vi "Initialize.vi"(7 "Serial Configuration":T1={"Baud Rate"=9600, "Parity"=0, "Data Bits"=8, "Stop Bits"=10, "Flow Control"=0} {"Flow Control" items=["None", "XON/XOFF", "RTS/CTS", "XON/XOFF & RTS/CTS", "DTR/DSR", "XON/XOFF & DTR/DSR"]; "Stop Bits" items=["1.0"=10, "1.5"=15, "2.0"=20]; "Data Bits" items=["7"=7, "8"=8]; "Parity" items=["None", "Odd", "Even", "Mark", "Space"]; "Baud Rate" items=["300"=300, "600"=600, "1200"=1200, "2400"=2400, "4800"=4800, "9600"=9600, "19200"=19200]}, 8 "error in (no error)":errorcluster, 9 "Reset (True)":bool=TRUE, 10 "ID Query (True)":bool=TRUE, 11 "VISA resource name":refnum<visa-resource-name>) -> (0 "error out":errorcluster, 3 "VISA resource name out":refnum<visa-resource-name>)   [LabVIEW 2012, in "Fluke 5080.lvlib"]
doc: "Establishes communication with the instrument and optionally performs an instrument identification query and/or an instrument reset. It also places the instrument in a default state needed for other instrument driver operations. Therefore, call this VI before calling other instrument driver VIs for this instrument. Generally, you need to call the Initialize VI only once at the beginning of an application."
uses:
  <instrlib>/Fluke 5080/Fluke 5080.lvlib
panel:
  # "(c) 2010 National Instruments.  ALL RIGHTS RESERVED."
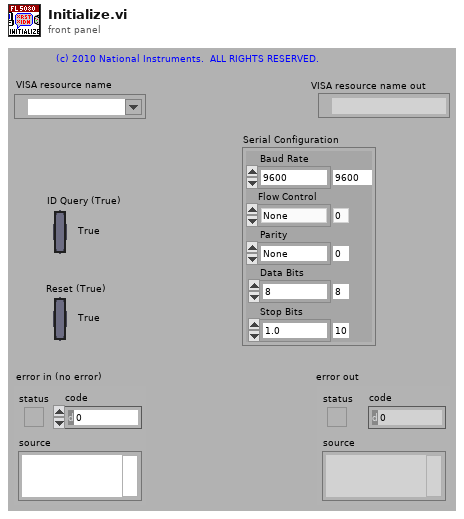
[diagram p1: front panel]
types:
  T1 = cluster{"Baud Rate":u32, "Parity":u16, "Data Bits":u16, "Stop Bits":u16, "Flow Control":u16}
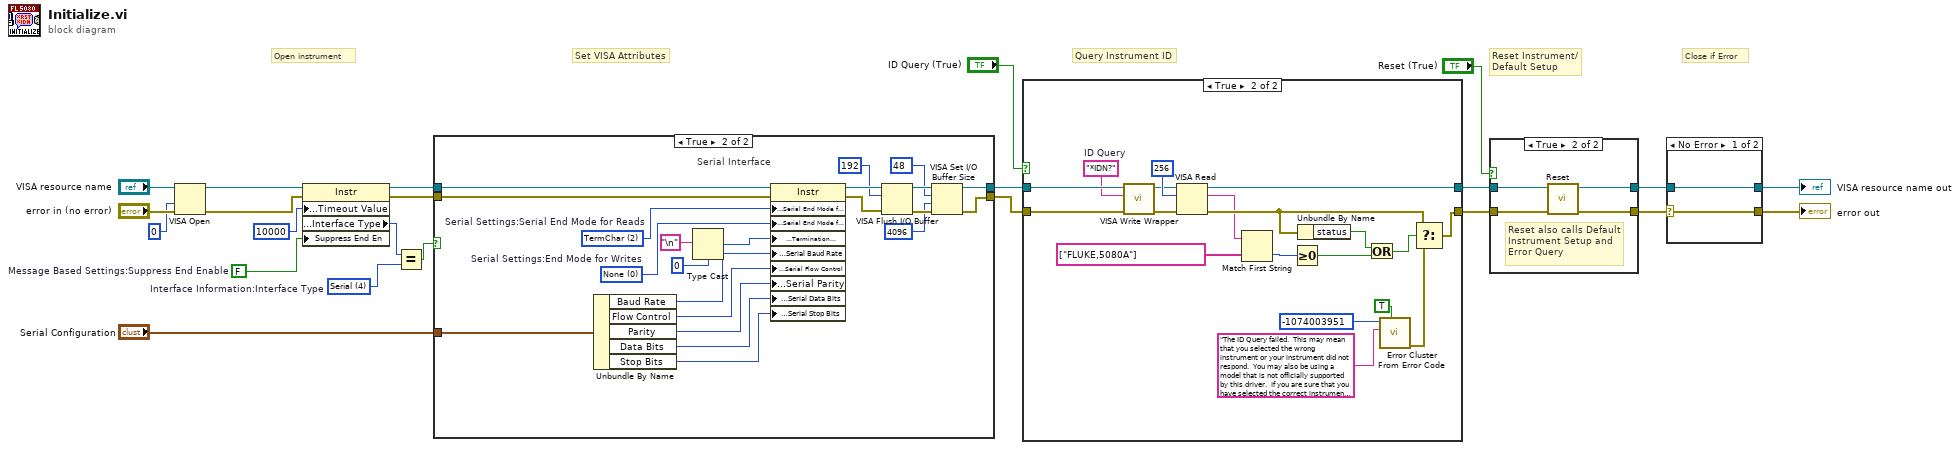
[diagram p0: block diagram]
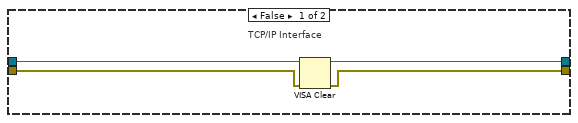
[diagram p2: hidden frame]
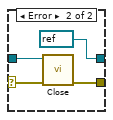
[diagram p3: hidden frame]
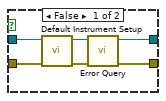
[diagram p4: hidden frame]
diagram:
  w3 = FALSE  # Message Based Settings:Suppress End Enable
  w12 = u16 4 items=["GPIB"=1, "VXI"=2, "GPIB-VXI"=3, "Serial"=4, "PXI"=5, "TCPIP"=6, "USB"=7]  # Interface Information:Interface Type
  # "Set VISA Attributes"
  # "Close if Error"
  # "Query Instrument ID"
  # "Reset Instrument/\nDefault Setup"
  # "Open instrument"
  n1 = VISA Open(access mode=u32 0, error in (no error)="error in (no error)", VISA resource name="VISA resource name") -> (VISA resource name=w5:refnum<visa-resource-name>, error out=w4:errorcluster)  [unwired: 2 out]
  n2 = property class="Instr"(reference=w5, error in=w4, "General Settings:Timeout Value"=u32 10000, "Suppress End En"=w3) -> (reference out=w15:refnum<visa-resource-name>, error out=w14:errorcluster, "Interface Information:Interface Type"=w19:u16)
  n3 = Equal?(x=w19, y=w12) -> (x = y?=w13:bool)
  n4 = case shown="True" w13 {
    tunnel: [w26 w46] -> w17
    tunnel: [w24 w43] -> w16
    tunnel: w15 -> [w27 w48]
    tunnel: w14 -> [w25 w49]
    tunnel: "Serial Configuration" -> [_ w33]
    frame False {
      # "TCP/IP Interface"
      n5 = VISA Clear(VISA resource name=w27, error in (no error)=w25) -> (VISA resource name out=w26:refnum<visa-resource-name>, error out=w24:errorcluster)
    }
    frame True {
      w29 = u16 0 items=["None", "Last Bit", "TermChar", "Break"]  # Serial Settings:End Mode for Writes
      w28 = u16 2 items=["None", "LastBit", "TermChar"]  # Serial Settings:Serial End Mode for Reads
      # "Serial Interface"
      n6 = Unbundle By Name(w33) -> ("Baud Rate"=w38:u32, "Flow Control"=w35:u16, "Parity"=w36:u16, "Data Bits"=w37:u16, "Stop Bits"=w34:u16)
      n7 = Type Cast(type=u8 0, x="\n") -> (*(type *) &x=w30:u8)
      n8 = property class="Instr"(reference=w48, error in=w49, "Serial Settings:Serial End Mode for Reads"=w28, "Serial Settings:Serial End Mode for Writes"=w29, "Message Based Settings:Termination Character"=w30, "Serial Settings:Serial Baud Rate"=w38, "Serial Settings:Serial Flow Control"=w35, "Serial Settings:Serial Parity"=w36, "Serial Settings:Serial Data Bits"=w37, "Serial Settings:Serial Stop Bits"=w34) -> (reference out=w42:refnum<visa-resource-name>, error out=w45:errorcluster)
      n9 = VISA Flush I/O Buffer(VISA resource name=w42, mask (16)=u16 192, error in (no error)=w45) -> (VISA resource name out=w47:refnum<visa-resource-name>, error out=w44:errorcluster)
      n10 = VISA Set I/O Buffer Size(VISA resource name=w47, mask (16)=u16 48, size (4096)=u32 4096 ("size (0)"), error in (no error)=w44) -> (VISA resource name out=w46:refnum<visa-resource-name>, error out=w43:errorcluster)
    }
  }
  n11 = case shown="True" "ID Query (True)" {
    tunnel: [w50 w70] -> w1
    tunnel: [w51 w69] -> w2
    tunnel: w17 -> [w51 w53]
    tunnel: w16 -> [w50 w54]
    frame False {
    }
    frame True {
      w52 = "*IDN?"  # ID Query
      n12 = call <instrlib>:"VISA Write Wrapper.vi"("error in (no error)"=w54, "Write Buffer"=w52, "VISA resource name"=w53) -> ("error out"=w55:errorcluster, "VISA resource name out"=w56:refnum<visa-resource-name>)  [unwired: 7 out]
      n13 = VISA Read(VISA resource name=w56, byte count=u32 256, error in (no error)=w55) -> (VISA resource name out=w69:refnum<visa-resource-name>, read buffer=w57:string, error out=w63:errorcluster)  [unwired: 1 out]
      n14 = Match First String(2:string[] ["FLUKE,5080A"], 3:w57) -> (0:w59:i32)  [unwired: 1 out]
      n15 = Greater Or Equal To 0?(x=w59) -> (x >= 0?=w61:bool)
      n16 = Unbundle By Name(w63) -> ("status"=w62:bool)
      n17 = Or(x=w62, y=w61) -> (x .or. y?=w60:bool)
      n18 = call <vilib>:"Error Cluster From Error Code.vi"("show call chain? (False)"=TRUE, "error message (\"\")"="The ID Query failed.  This may mean that you selected the wrong instrument or your instrument did not respond.  You may also be using a model that is not officially supported by this driver.  If you are sure that you have selected the correct instrument and it is responding, try disabling the ID Query." ("Source (VI Name)"), "error code (0)"=-1074003951 ("Code")) -> ("error out"=w67:errorcluster)  [unwired: 1 in, 5 out]
      n19 = Select(t=w63, s=w60, f=w67) -> (s? t:f=w70:errorcluster)
    }
  }
  n20 = case shown="True" "Reset (True)" {
    tunnel: w1 -> [w75 w77]
    tunnel: [w72 w80] -> w7
    tunnel: w2 -> [w76 w78]
    tunnel: [w73 w79] -> w8
    frame False {
      n21 = call <instrlib>:"Default Instrument Setup.vi"("error in (no error)"=w75, "VISA resource name"=w76) -> ("error out"=w71:errorcluster, "VISA resource name out"=w74:refnum<visa-resource-name>)  [unwired: 8 out]
      n22 = call <instrlib>:"Error Query.vi"("error in (no error)"=w71, "VISA resource name"=w74) -> ("error out"=w72:errorcluster, "VISA resource name out"=w73:refnum<visa-resource-name>)  [unwired: 8 out]
    }
    frame True {
      # "Reset also calls Default Instrument Setup and Error Query"
      n23 = call <instrlib>:"Reset.vi"("error in (no error)"=w77, "VISA resource name"=w78) -> ("error out"=w80:errorcluster, "VISA resource name out"=w79:refnum<visa-resource-name>)  [unwired: 8 out]
    }
  }
  n24 = case shown="No Error" w7 {
    selector: w7 -> [w81 w84]
    tunnel: w8 -> [w82 w85]
    tunnel: [w82 refnum<visa-resource-name> refnum ("VISA resource name out")] -> w10
    tunnel: [w81 w86] -> w9
    frame No Error {
    }
    frame Error {
      n25 = call <instrlib>:"Close.vi"("error in (no error)"=w84, "VISA resource name"=w85) -> ("error out"=w86:errorcluster)  [unwired: 9 out]
    }
  }
  "VISA resource name out" <- w10
  "error out" <- w9
